vi "notify_with_timeout_v1.0.vi"(9 "blink_timer(sec)":dbl=0.5, 10 "timer(sec)":dbl=3.0, 11 "message in":string="Not valid to run the test..") -> ()   [LabVIEW 2025]
doc: "Use this template to build a producer/consumer design pattern with events to produce queue items. Use this design pattern instead of the User Interface Event Handler pattern for user interfaces when you want to execute code asynchronously in response to an event without slowing the user interface responsiveness."
uses:
  <vilib>/Utility/error.llb/Trim Whitespace One-Sided.vi
panel:
  out "consumer_exit":bool
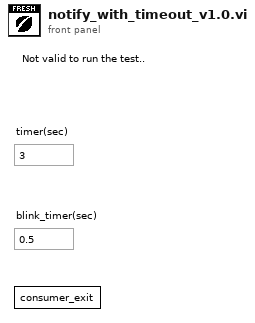
[diagram p1: front panel]
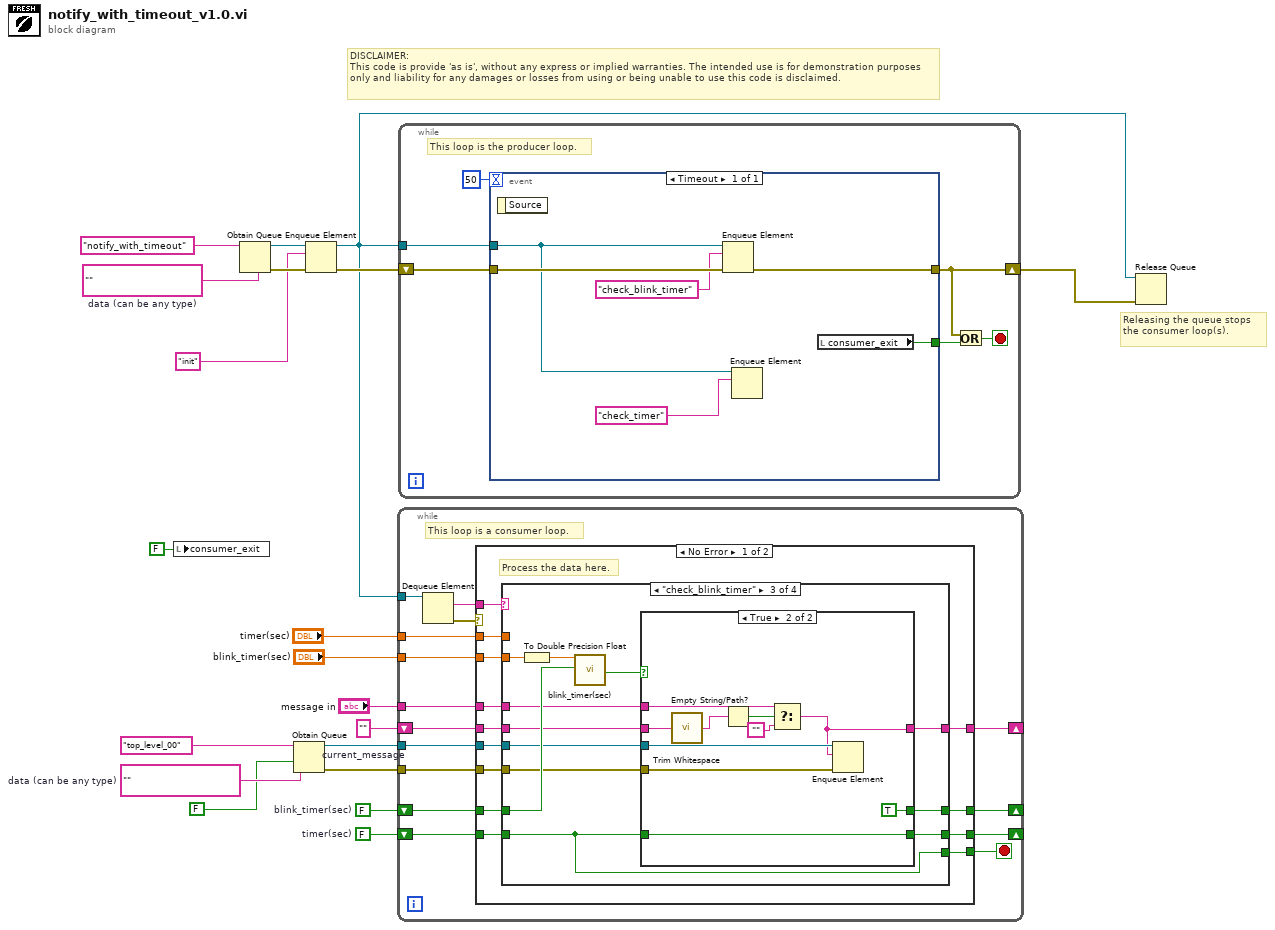
[diagram p0: block diagram]
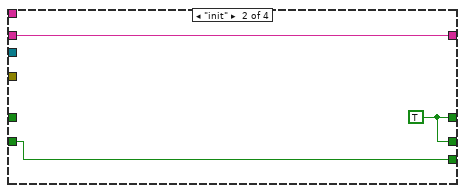
[diagram p3: hidden frame]
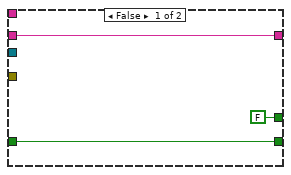
[diagram p4: hidden frame]
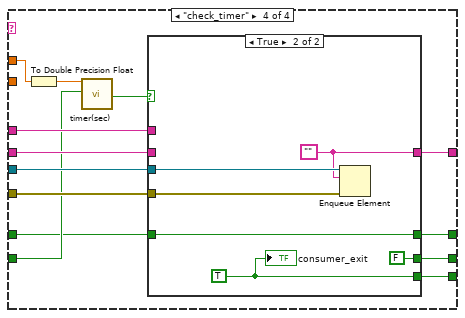
[diagram p5: hidden frame]
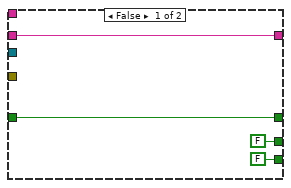
[diagram p6: hidden frame]
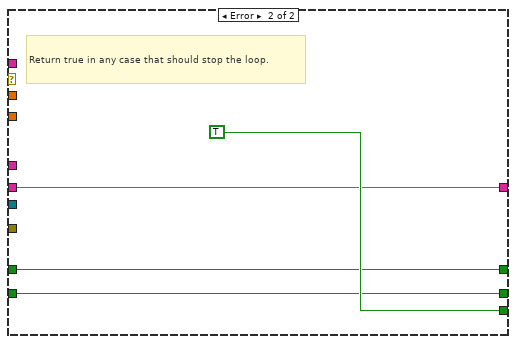
[diagram p7: hidden frame]
diagram:
  w12 = ""  # current_message
  w9 = FALSE  # timer(sec)
  w15 = FALSE  # blink_timer(sec)
  w17 = ""  # data (can be any type)
  w19 = ""  # data (can be any type)
  # "DISCLAIMER:\nThis code is provide 'as is', without any express or implied warranties. The intended use is for demonstration purposes only and liability for any damages or losses from using or being unable to use this code is disclaimed."
  # "Releasing the queue stops the consumer loop(s)."
  n1 = local write "consumer_exit"(FALSE ("consumer_exit")) -> ()
  n2 = Obtain Queue(name (unnamed)="notify_with_timeout", element data type=w19) -> (queue out=w6:refnum<queue>, error out=w8:errorcluster)  [unwired: 3 in, 1 out]
  n3 = Obtain Queue(name (unnamed)="top_level_00", element data type=w17, create if not found? (T)=FALSE) -> (queue out=w16:refnum<queue>, error out=w10:errorcluster)  [unwired: 2 in, 1 out]
  n4 = Enqueue Element(queue=w6, element="init", error in (no error)=w8) -> (queue out=w5:refnum<queue>, error out=w7:errorcluster)  [unwired: 1 in, 1 out]
  n5 = while {
    tunnel: w5 -> [w35]
    tunnel: w16 -> [w28]
    shift-right: [w30] -> _
    shift-left: w15 -> [w31]
    tunnel: "blink_timer(sec)" -> [w29]
    shift-right: [w24] -> _
    shift-left: w12 -> [w27]
    tunnel: "message in" -> [w26]
    tunnel: w10 -> [w25]
    shift-right: [w22] -> _
    shift-left: w9 -> [w23]
    tunnel: "timer(sec)" -> [w21]
    stop <- w32 stop-if-true
    # "This loop is a consumer loop."
    n6 = Dequeue Element(queue=w35) -> (element=w33:string, error out=w34:errorcluster)  [unwired: 2 in, 2 out]
    n7 = case shown="No Error" w34 {
      tunnel: w33 -> [w48 _]
      tunnel: [w36 TRUE] -> w32
      tunnel: w31 -> [w47 w103]
      tunnel: [w46 w103] -> w30
      tunnel: w29 -> [w45 _]
      tunnel: w28 -> [w44 _]
      tunnel: w27 -> [w43 w102]
      tunnel: w26 -> [w42 _]
      tunnel: w25 -> [w41 _]
      tunnel: [w40 w102] -> w24
      tunnel: w23 -> [w39 w104]
      tunnel: [w38 w104] -> w22
      tunnel: w21 -> [w37 _]
      frame No Error {
        # "Process the data here."
        n8 = case shown="\"check_blink_timer\"" w48 {
          tunnel: w47 -> [_ _ w65 w80]
          tunnel: [_ w52 w58 w85] -> w46
          tunnel: w45 -> [_ _ w64 _]
          tunnel: w44 -> [_ _ w62 w89]
          tunnel: w43 -> [w50 w53 w61 w88]
          tunnel: w42 -> [_ _ w60 w87]
          tunnel: w41 -> [_ _ w59 w86]
          tunnel: [w50 w53 w57 w84] -> w40
          tunnel: w39 -> [w49 w51 w56 w81]
          tunnel: [w49 w52 w55 w83] -> w38
          tunnel: w37 -> [_ _ _ w82]
          tunnel: [w49 w51 w56 w79] -> w36
          frame Default {
          }
          frame "init" {
            w52 = TRUE
          }
          frame "check_blink_timer" {
            n9 = To Double Precision Float(number=w64) -> (double precision float=w63:dbl)
            n10 = call "blink_timer(sec)"("Time Target (s)"=w63, "Reset"=w65) -> ("Time has Elapsed"=w54:bool)  [unwired: 10 in, 7 out]
            n11 = case shown="True" w54 {
              tunnel: w62 -> [_ w78]
              tunnel: w61 -> [w67 w77]
              tunnel: w60 -> [_ w75]
              tunnel: w59 -> [_ w73]
              tunnel: [FALSE TRUE] -> w58
              tunnel: [w67 w71] -> w57
              tunnel: w56 -> [w66 w70]
              tunnel: [w66 w70] -> w55
              frame False {
              }
              frame True {
                n12 = call <vilib>:"Trim Whitespace.vi"("string"=w77) -> ("trimmed string"=w74:string)  [unwired: 1 in]
                n13 = Empty String/Path?(string/path=w74) -> (empty?=w76:bool)
                n14 = Select(t=w75, s=w76, f="") -> (s? t:f=w71:string)
                n15 = Enqueue Element(queue=w78, element=w71, error in (no error)=w73) -> ()  [unwired: 1 in, 3 out]
              }
            }
          }
          frame "check_timer" {
            n16 = To Double Precision Float(number=w82) -> (double precision float=w91:dbl)
            n17 = call "timer(sec)"("Time Target (s)"=w91, "Reset"=w81) -> ("Time has Elapsed"=w90:bool)  [unwired: 10 in, 7 out]
            n18 = case shown="True" w90 {
              tunnel: w89 -> [_ w101]
              tunnel: w88 -> [w95 _]
              tunnel: w87 -> [_ _]
              tunnel: w86 -> [_ w100]
              tunnel: [w94 w99] -> w85
              tunnel: [w95 w97] -> w84
              tunnel: [FALSE ("timer(sec)") FALSE ("timer(sec)")] -> w83
              tunnel: w80 -> [w94 w99]
              tunnel: [FALSE ("timer(sec)") w96] -> w79
              frame False {
              }
              frame True {
                w96 = TRUE ("timer(sec)")
                w97 = ""
                n19 = Enqueue Element(queue=w101, element=w97, error in (no error)=w100) -> ()  [unwired: 1 in, 3 out]
                "consumer_exit" <- w96
              }
            }
          }
        }
      }
      frame Error {
        # "Return true in any case that should stop the loop."
      }
    }
  }
  n20 = while {
    shift-right: [w107] -> w20
    shift-left: w7 -> [w110]
    tunnel: w5 -> [w111]
    stop <- w108 stop-if-true
    # "This loop is the producer loop."
    n21 = event shown="[0] Timeout" {
      selector: _ -> [_]
      dyn-events: _ -> [_]
      timeout: 50 -> [_]
      tunnel: w111 -> [w113]
      tunnel: w110 -> [w117]
      tunnel: [w112] -> w107
      tunnel: [w114] -> w109
      event Timeout {
        n22 = event-data() -> ()  [unwired: 1 in, 1 out]
        n23 = Enqueue Element(queue=w113, element="check_blink_timer", error in (no error)=w117) -> (error out=w112:errorcluster)  [unwired: 1 in, 2 out]
        n24 = Enqueue Element(queue=w113, element="check_timer") -> ()  [unwired: 2 in, 3 out]
        n25 = local read "consumer_exit"() -> (w114:bool)
      }
    }
    n26 = Or(x=w107, y=w109) -> (x .or. y?=w108:bool)
  }
  n27 = Release Queue(queue=w5, error in (no error)=w20) -> ()  [unwired: 1 in, 3 out]
